vi "题目一.vi"   [LabVIEW 2017]
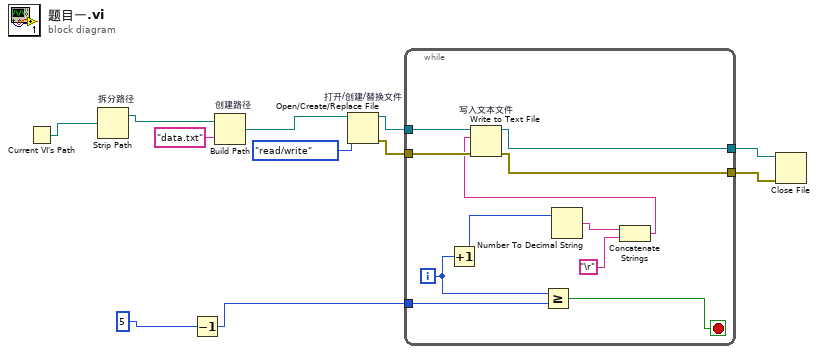
[diagram p0: block diagram]
diagram:
  n1 = Current VI's Path() -> (path=w8:path)
  n2 = Strip Path "拆分路径"(path=w8) -> (stripped path=w7:path)  [unwired: 1 out]
  n3 = Decrement(x=5) -> (x-1=w4:i32)
  n4 = Build Path "创建路径"(base path=w7, name or relative path="data.txt" ("名称或相对路径")) -> (appended path=w11:path)
  n5 = Open/Create/Replace File "打开/创建/替换文件"(file path (use dialog)=w11, access (0:read/write)=enum16{"read/write", "read-only", "write-only"}."read/write" ("权限(0:read/write)")) -> (refnum out=w10:refnum<file>, error out=w3:errorcluster)  [unwired: 4 in, 1 out]
  n6 = while {
    tunnel: w10 -> [w22]
    tunnel: w4 -> [w21]
    tunnel: w3 -> [w20]
    tunnel: [w13] -> w2
    tunnel: [w12] -> w1
    i -> [w16]
    stop <- w15 stop-if-true
    n7 = Increment(x=w16) -> (x+1=w19:i32)
    n8 = Greater Or Equal?(x=w16, y=w21) -> (x >= y?=w15:bool)
    n9 = Number To Decimal String(number=w19) -> (decimal integer string=w18:string)  [unwired: 1 in]
    n10 = Concatenate Strings(w18, "\r") -> (w17:string)
    n11 = Write to Text File "写入文本文件"(file (use dialog)=w22, text=w17, error in=w20) -> (refnum out=w12:refnum<file>, error out=w13:errorcluster)  [unwired: 1 in, 1 out]
  }
  n12 = Close File(refnum=w1, error in=w2) -> ()  [unwired: 2 out]
